vi "Neko.vi"() -> ()   [LabVIEW 2020]
panel:
  out "Vertical":i32
  out "Horizontal":i32
  out "Ring":u16(ring)
  in  "stop":bool
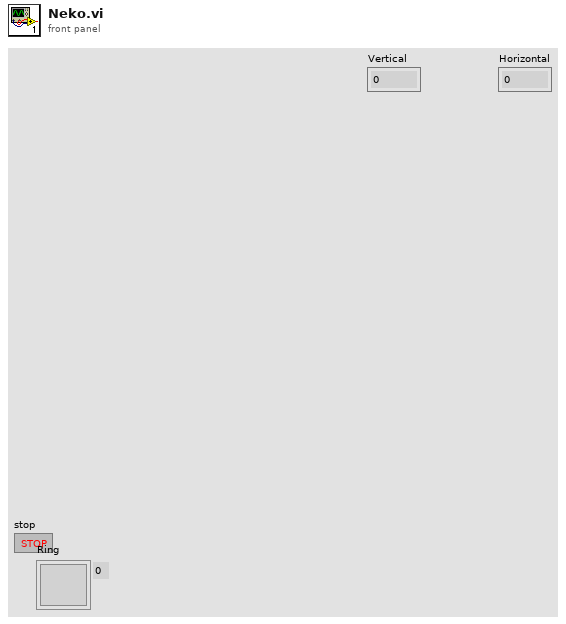
[diagram p1: front panel]
types:
  T1 = typedef "LVPoint32TypeDef.ctl" = cluster{"Horizontal":i32, "Vertical":i32}
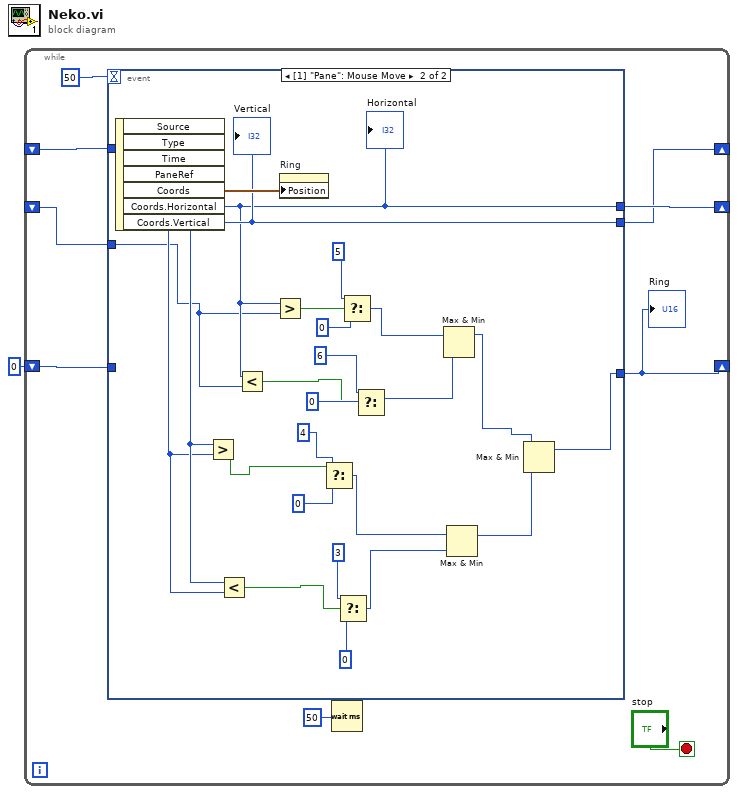
[diagram p0: block diagram]
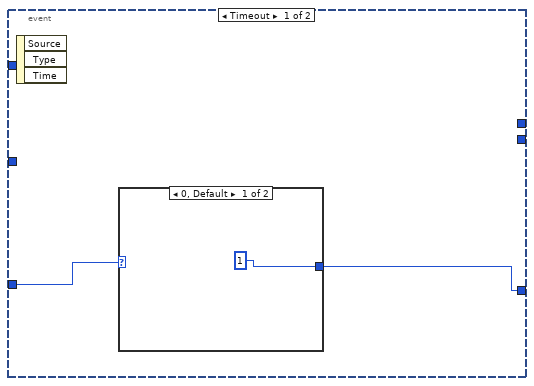
[diagram p2: hidden frame]
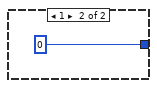
[diagram p3: hidden frame]
diagram:
  n1 = while {
    shift-right: [w2] -> _
    shift-left: 0 -> [w8]
    shift-right: [w6] -> _
    shift-left: _ -> [w5]
    shift-right: [w4] -> _
    shift-left: _ -> [w3]
    stop <- "stop" stop-if-true
    n2 = event shown="[1] \"Pane\": Mouse Move" {
      selector: _ -> [_ _]
      dyn-events: _ -> [_ _]
      timeout: 50 -> [_ _]
      tunnel: w8 -> [w12 _]
      tunnel: [_ w16] -> w6
      tunnel: w5 -> [_ w15]
      tunnel: [_ w25] -> w4
      tunnel: w3 -> [_ w24]
      tunnel: [w11 w17] -> w2
      event Timeout {
        n3 = event-data() -> ()  [unwired: 1 in, 3 out]
        n4 = case shown="0, Default" w12 {
          tunnel: [1 0] -> w11
          frame 0, Default {
          }
          frame 1 {
          }
        }
      }
      event Mouse Move {
        n5 = event-data() -> ("Coords"=w38:T1, "Coords.Horizontal"=w16:i32, "Coords.Vertical"=w25:i32)  [unwired: 1 in, 4 out]
        "Horizontal" <- w16
        "Vertical" <- w25
        n6 = Greater?(x=w25, y=w24) -> (0:w34:bool)
        n7 = Less?(x=w25, y=w24) -> (x < y?=w27:bool)
        n8 = Less?(x=w16, y=w15) -> (x < y?=w30:bool)
        n9 = Greater?(x=w16, y=w15) -> (0:w37:bool)
        n10 = property on="Ring" class="Ring (strict)"("Position"=w38) -> ()  [unwired: 2 in, 2 out]
        n11 = Select(t=4, s=w34, f=0) -> (s? t:f=w21:i32)
        n12 = Select(t=3, s=w27, f=0) -> (s? t:f=w20:i32)
        n13 = Select(t=5, s=w37, f=0) -> (s? t:f=w23:i32)
        n14 = Select(t=6, s=w30, f=0) -> (s? t:f=w22:i32)
        n15 = Max & Min(x=w23, y=w22) -> (max(x,y)=w19:i32)  [unwired: 1 out]
        n16 = Max & Min(x=w21, y=w20) -> (max(x,y)=w18:i32)  [unwired: 1 out]
        n17 = Max & Min(x=w19, y=w18) -> (max(x,y)=w17:i32)  [unwired: 1 out]
      }
    }
    "Ring" <- w2
    n18 = Wait (ms)(milliseconds to wait=50) -> ()  [unwired: 1 out]
  }
